vi "KFStage.vi"(6 "Initial condition":cluster{"H0":dbl, "xd0":dbl, "D0":dbl}={"H0"=4.55, "xd0"=0.275, "D0"=4.2}, 8 "error in (no error)":errorcluster, 9 "delta_t":dbl, 10 "NoiseVariance":dbl, 11 "Synx":cdb[][](array[numeric])) -> (0 "error out":errorcluster, 1 "KalmanGain":dbl[][](array[numeric]), 2 "Pk":dbl[][](array[numeric]), 3 "xk":dbl[][](array[numeric]))   [LabVIEW 2014, in "AppPlugins.lvlib" / "ModelValidationPlugin.lvclass"]
uses:
  ModelValidationPlugin.lvclass
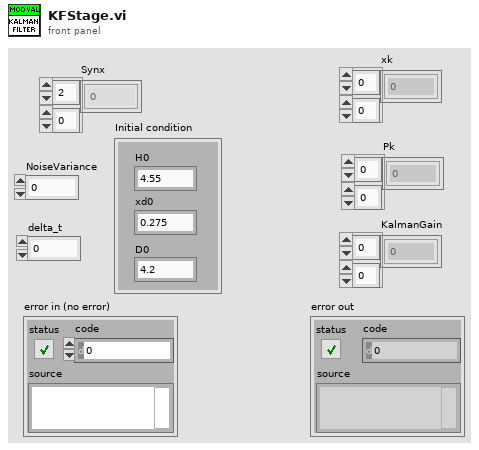
[diagram p1: front panel]
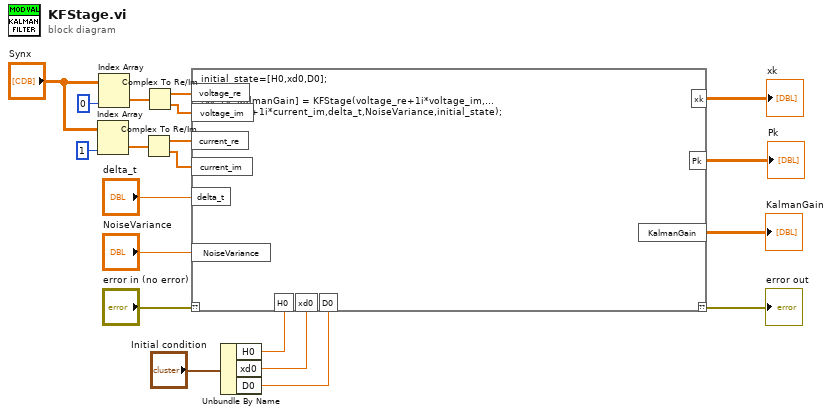
[diagram p0: block diagram]
diagram:
  n1 = Index Array(array="Synx", index (col)=1) -> (element=w9:cdb[])  [unwired: 1 in]
  n2 = Index Array(array="Synx", index (col)=0 ("disabled index (col)")) -> (element=w10:cdb[])  [unwired: 1 in]
  n3 = Complex To Re/Im(x + iy=w9) -> (x=w6:dbl[], y=w5:dbl[])
  n4 = Complex To Re/Im(x + iy=w10) -> (x=w7:dbl[], y=w8:dbl[])
  n5 = Unbundle By Name("Initial condition") -> ("H0"=w3:dbl, "xd0"=w2:dbl, "D0"=w1:dbl)
  n6 = script code="initial_state=[H0,xd0,D0];\n\n[xk, Pk, KalmanGain] = KFStage(voltage_re+1i*voltage_im,...\ncurrent_re+1i*current_im,delta_t,NoiseVariance,initial_state);"("??"="error in (no error)", "voltage_re"=w7, "delta_t"="delta_t", "NoiseVariance"="NoiseVariance", "current_re"=w6, "voltage_im"=w8, "current_im"=w5, "H0"=w3, "xd0"=w2, "D0"=w1) -> ("??"=→"error out":errorcluster, "xk"=→"xk":dbl[][], "KalmanGain"=→"KalmanGain":dbl[][], "Pk"=→"Pk":dbl[][])
